vi "Tosca-Create Digital Outputs.vi"(6 "Rep trigger only?":bool, 7 "Trial start? (F)":bool, 8 "error in (no error)":errorcluster, 10 "DO":T1) -> (0 "error out":errorcluster, 3 "DO Array":bool[][](array[boolean]))   [LabVIEW 2020]
uses:
  Typedefs/Tosca-DO Runtime.ctl
panel:
  out "Waveform Graph":i16[][](graph)
  in  "Pulse width (us)":dbl=20000.0
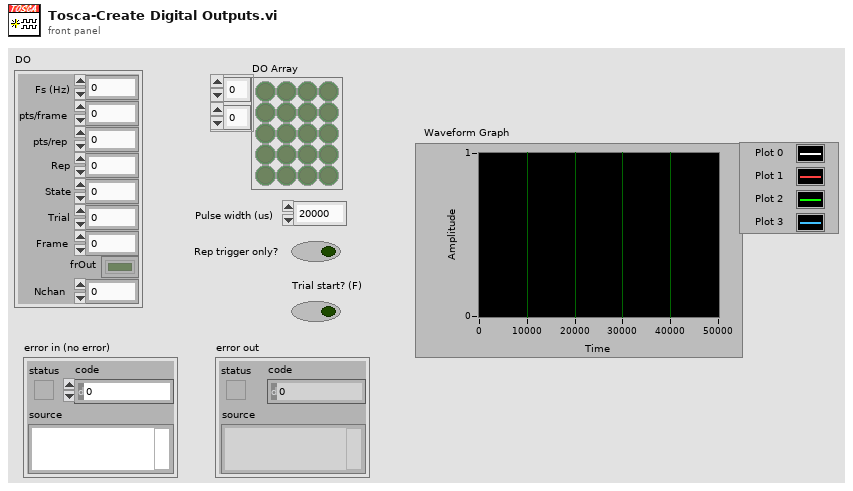
[diagram p1: front panel]
types:
  T1 = typedef "Tosca-DO Runtime.ctl" = cluster{"Fs (Hz)":dbl, "pts/frame":i32, "pts/rep":i32, "Rep":i32, "State":i32, "Trial":i32, "Frame":i32, "frOut":bool[], "Nchan":i32}
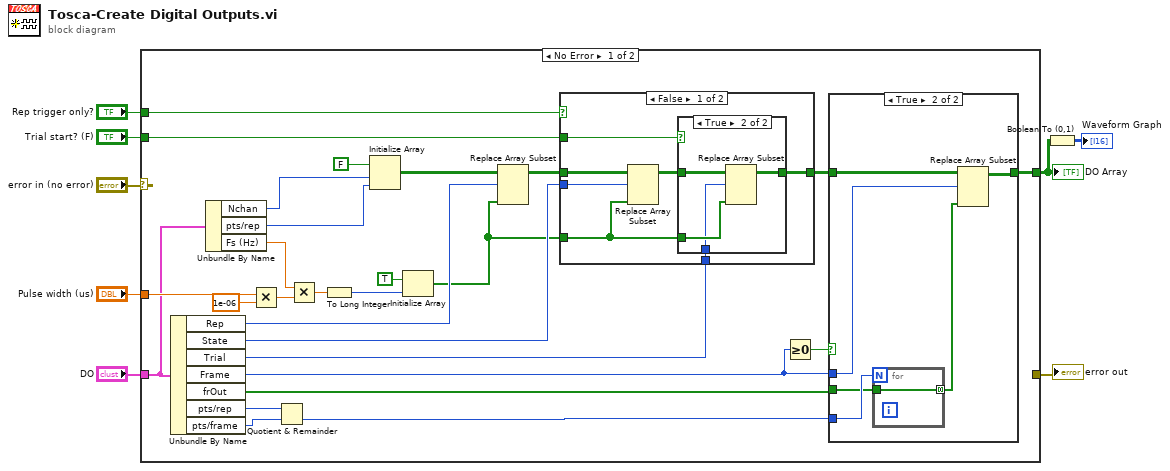
[diagram p0: block diagram]
diagram:
  n1 = case shown="No Error" "error in (no error)" {
    selector: "error in (no error)" -> [_ w57]
    tunnel: "Rep trigger only?" -> [w24 _]
    tunnel: [w17 _] -> w4
    tunnel: "Pulse width (us)" -> [w33 _]
    tunnel: [_ w57] -> w5
    tunnel: "Trial start? (F)" -> [w26 _]
    tunnel: "DO" -> [w12 _]
    frame No Error {
      n2 = Unbundle By Name(w12) -> ("Rep"=w21:i32, "State"=w20:i32, "Trial"=w19:i32, "Frame"=w16:i32, "frOut"=w14:bool[], "pts/rep"=w11:i32, "pts/frame"=w10:i32)
      n3 = Unbundle By Name(w12) -> ("Nchan"=w27:i32, "pts/rep"=w35:i32, "Fs (Hz)"=w31:dbl)
      n4 = Multiply(x=w33, y=1e-06) -> (x*y=w30:dbl)
      n5 = Quotient & Remainder(x=w11, y=w10) -> (floor(x/y)=w9:i32)  [unwired: 1 out]
      n6 = Multiply(x=w31, y=w30) -> (x*y=w29:dbl)
      n7 = To Long Integer(number=w29) -> (32bit integer=w28:i32)
      n8 = Initialize Array(FALSE, w27, w35) -> (w23:bool[][])
      n9 = Initialize Array(TRUE, w28) -> (w13:bool[])
      n10 = Replace Array Subset(array=w23, new element=w13, index (row)=w21) -> (w22:bool[][])  [unwired: 1 in]
      n11 = case shown="False" w24 {
        tunnel: w22 -> [w50 w56]
        tunnel: [w48 w56] -> w18
        tunnel: w26 -> [w47 _]
        tunnel: w13 -> [w46 _]
        tunnel: w20 -> [w45 _]
        tunnel: w19 -> [w44 _]
        frame False {
          n12 = Replace Array Subset(array=w50, new element=w46, index (row)=w45) -> (w49:bool[][])  [unwired: 1 in]
          n13 = case shown="True" w47 {
            tunnel: w49 -> [w51 w55]
            tunnel: [w51 w54] -> w48
            tunnel: w46 -> [_ w53]
            tunnel: w44 -> [_ w52]
            frame False {
            }
            frame True {
              n14 = Replace Array Subset(array=w55, new element=w53, index (row)=w52) -> (w54:bool[][])  [unwired: 1 in]
            }
          }
        }
        frame True {
        }
      }
      n15 = Greater Or Equal To 0?(x=w16) -> (x >= 0?=w15:bool)
      n16 = case shown="True" w15 {
        tunnel: w18 -> [w36 w42]
        tunnel: [w36 w41] -> w17
        tunnel: w16 -> [_ w40]
        tunnel: w14 -> [_ w38]
        tunnel: w9 -> [_ w39]
        frame False {
        }
        frame True {
          n17 = for {
            N: w39 -> [_]
            tunnel: w38 -> [w43]
            tunnel: [w43] -> w37 mode=concatenating
          }
          n18 = Replace Array Subset(array=w42, new element=w37, index (row)=w40) -> (w41:bool[][])  [unwired: 1 in]
        }
      }
    }
    frame Error {
    }
  }
  "error out" <- w5
  "DO Array" <- w4
  n19 = Boolean To (0,1)(Boolean=w4) -> (0, 1=→"Waveform Graph":i16[][])
